vi "Regiter Event Callback.vi"(8 "error in (no error)":errorcluster, 10 "customData":u32, 11 "pEventCallbackProc":cluster{}) -> (0 "error out":errorcluster, 2 "customData out":u32, 3 "function return":i32)   [LabVIEW 2017, in "imgAcquisition.lvlib"]
doc: "DLLFunction int __stdcall ImageCapRegiterEventCallback(pEventCallback pEventCallbackProc, void* customData=NULL);"
uses:
  imgAcquisition.lvlib
  lib/ImageCaptureDLL.dll
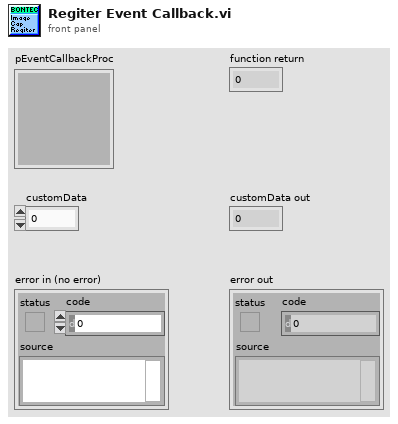
[diagram p1: front panel]
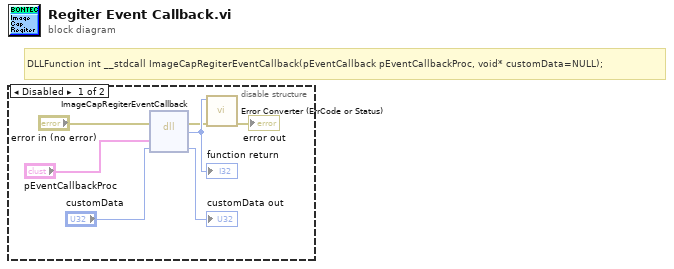
[diagram p0: block diagram]
diagram:
  # "DLLFunction int __stdcall ImageCapRegiterEventCallback(pEventCallback pEventCallbackProc, void* customData=NULL);"
  n1 = disable-structure shown="Disabled" {
    frame Disabled {
      n2 = dll-call lib="F:/BonTechFlatPanelLVDriver/lib/ImageCaptureDLL.*" fn="ImageCapRegiterEventCallback"(error in="error in (no error)", "pEventCallbackProc"="pEventCallbackProc", "customData"="customData") -> (error out=w2:errorcluster, w7:i32, "customData"=→"customData out":u32)  [unwired: 3 in, 1 out]
      "function return" <- w7
      n3 = call "Error Converter (ErrCode or Status).vi"("error in (no error)"=w2, "error code"=w7) -> ("error out"=→"error out":errorcluster)  [unwired: 9 in]
    }
    frame Enabled {
    }
  }
